vi "MT Generate PSK Synchronization Parameters (bit array).vi"(0 "PSK system parameters":T1={"samples per symbol (16)"=16, "symbol map"=[], "differential PSK"=enum."disable", "PSK type"=0} {"PSK type" items=["normal", "shifted", "offset"]; "symbol map" format="%.3f"}, 5 "sync bits":i8[](array[numeric]), 11 "error in (no error)":errorcluster, 12 "expected sync location (symbols)":i32=-1, 13 "sync location uncertainty (symbols)":i32=10, 14 "sync indent (symbols)":i32) -> (4 "PSK synchronization parameters":T2 {"sync sequence" format="%.2f"}, 15 "error out":errorcluster)   [LabVIEW 2020, in "niDMT.lvlib"]
doc: "This polymorphic instance generates synchronization parameters for PSK demodulation using a synchronization sequence directly represented by the <B>sync bits</B> array."
uses:
  <vilib>/addons/Modulation/niDMT.lvlib
  <vilib>/addons/Modulation/niAMT.lvlib
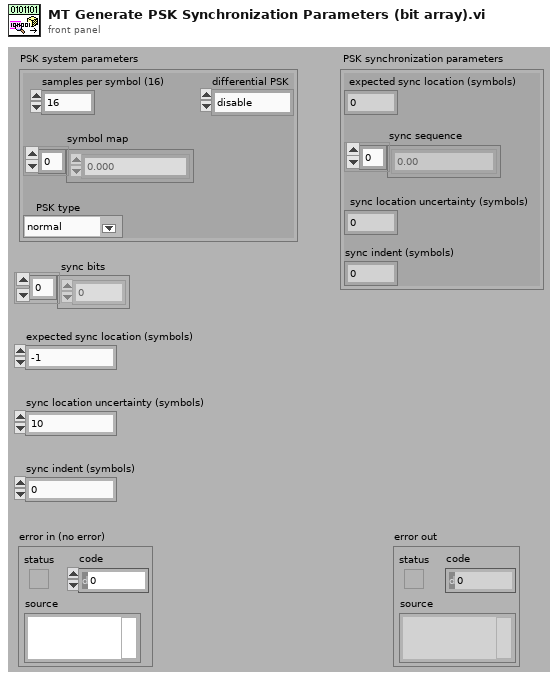
[diagram p1: front panel]
types:
  T1 = cluster{"samples per symbol (16)":i32, "symbol map":cdb[], "differential PSK":enum16{"disable", "enable"}, "PSK type":u16}
  T2 = cluster{"expected sync location (symbols)":i32, "sync sequence":cdb[], "sync location uncertainty (symbols)":i32, "sync indent (symbols)":i32}
  T3 = typedef "niDMT.lvlib/PSK Sync Parameters.ctl" = cluster{"expected sync location (symbols)":i32, "sync sequence":cdb[], "sync location uncertainty (symbols)":i32, "sync indent (symbols)":i32}
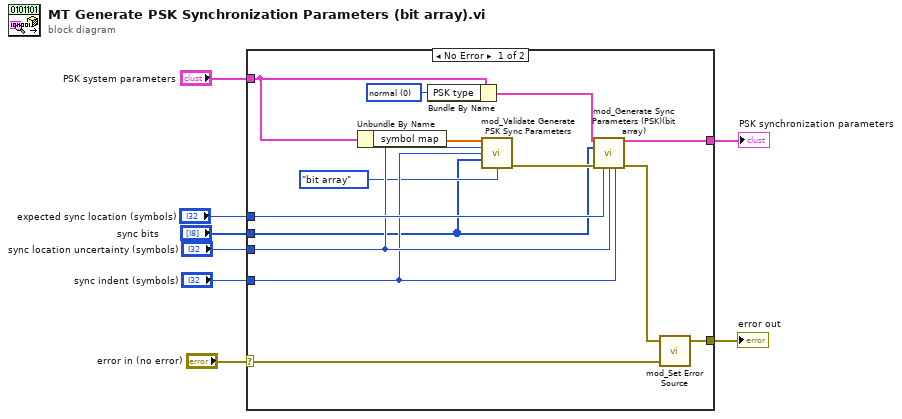
[diagram p0: block diagram]
diagram:
  n1 = case shown="No Error" "error in (no error)" {
    selector: "error in (no error)" -> [w21 w23]
    tunnel: [w18 _] -> w8
    tunnel: "expected sync location (symbols)" -> [w20 _]
    tunnel: "sync location uncertainty (symbols)" -> [w15 _]
    tunnel: "sync indent (symbols)" -> [w14 _]
    tunnel: "sync bits" -> [w12 _]
    tunnel: [w22 w23] -> w2
    tunnel: "PSK system parameters" -> [w11 _]
    frame No Error {
      w9 = u16 0 items=["normal", "shifted", "offset"] ("PSK type")
      n2 = Unbundle By Name(w11) -> ("symbol map"=w16:cdb[])
      n3 = Bundle By Name(cluster=w11, "PSK type"=w9) -> (w10:T1)
      n4 = call <vilib>:"mod_Validate Generate PSK Sync Parameters.vi"("symbol map"=w16, "sync location uncertainty (symbols)"=w15, "sync indent (symbols)"=w14, "sync bits"=w12, "sync bits specification"=enum16{"bit array", "number array", "number"}."bit array") -> ("error out"=w17:errorcluster)  [unwired: 2 in, 8 out]
      n5 = call <vilib>:"mod_Generate Sync Parameters (PSK)(bit array).vi"("PSK system parameters"=w10, "sync bits"=w12, "error in (no error)"=w17, "expected sync location (symbols)"=w20, "sync location uncertainty (symbols)"=w15, "sync indent (symbols)"=w14) -> ("PSK synchronization parameters"=w18:T3, "error out"=w19:errorcluster)  [unwired: 8 out]
      n6 = call <vilib>:"mod_Set Error Source.vi"("initial error in (no error)"=w21, "final error in (no error)"=w19) -> ("error out"=w22:errorcluster)  [unwired: 3 out]
    }
    frame Error {
    }
  }
  "PSK synchronization parameters" <- w8
  "error out" <- w2
